vi "XY Graph Data Types.vi"() -> ()   [LabVIEW 2023]
doc: "Illustrates the various data types that the XY Graph accepts. Use the XY Graph to display data that is not uniformly distributed along the X-axis. This is particularly useful when displaying data that was sampled at a variable rate. The XY Graph is also useful for displaying data that is formatted as (X,Y) pairs."
panel:
  in  "Tab Control":T1(tab)
  out "Single Plot (Array of X,Y Pairs)":cluster{i32, dbl}[](graph)
  out "Multiple Plots (Array of X,Y Pairs)":cluster{cluster{i32, dbl}[]}[](graph)
  out "Single Plot (X Array and Y Array)":cluster{i32[], dbl[]}(graph)
  out "Multiple Plots (X Array and Y Array)":cluster{i32[], dbl[]}[](graph)
  # "Overview: Demonstrates various XY Graph data types.\nInstructions:\n1. Run the VI.\n2. Switch between the tabs to observe the appearance of the various XY Graphs."
  # "XY graphs that use (X,Y) pairs are arrays of clusters on the block diagram."
  # "XY graphs that use arrays of X values and arrays of Y values are clusters of arrays on the block diagram."
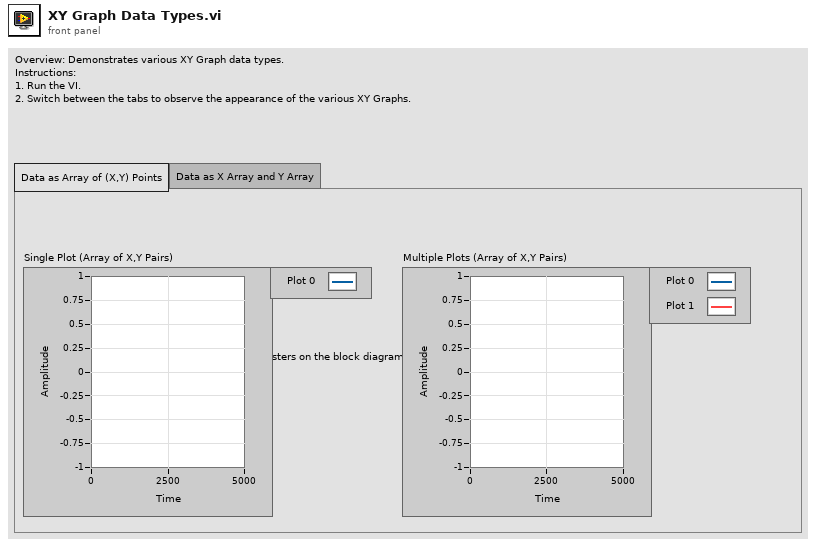
[diagram p1: front panel]
types:
  T1 = enum32{"Data as Array of (X,Y) Points", "Data as X Array and Y Array"}
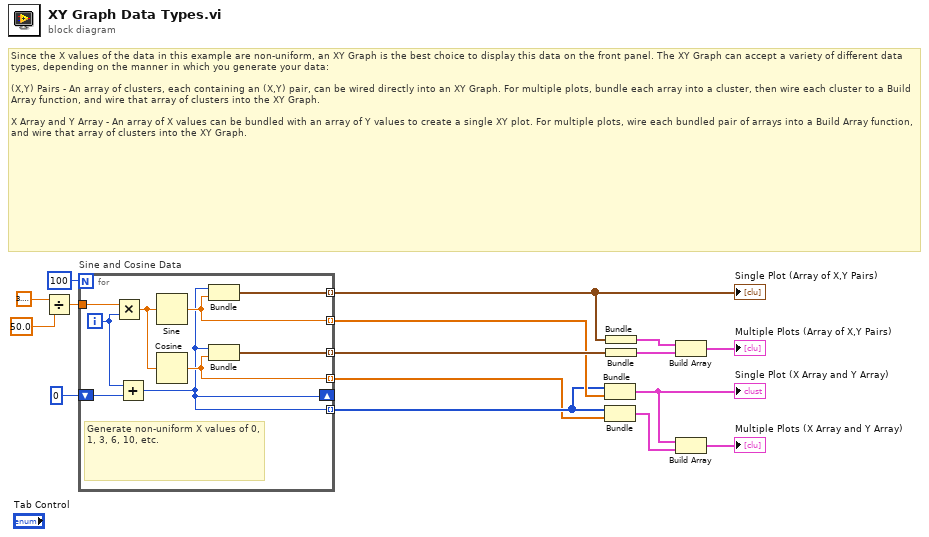
[diagram p0: block diagram]
diagram:
  # "Since the X values of the data in this example are non-uniform, an XY Graph is the best choice to display this data on the front panel. The XY Graph can accept a variety of different data types, depending on the manner in which you generate your data:\n\n(X,Y) Pairs - An array of clusters, each containing an (X,Y) pair, can be wired directly into an XY Graph. For multiple plots, bundle each array into a cluster, then wire each cluster to a Build Array function, and wire that array of clusters into the XY Graph.\n\nX Array and Y Array - An array of X values can be bundled with an array of Y values to create a single XY plot. For multiple plots, wire each bundled pair of arrays into a Build Array function, and wire that array of clusters into the XY Graph."
  n1 = Divide(x=3.141592653589793, y=50.0) -> (x/y=w14:dbl)
  n2 = for "Sine and Cosine Data" {
    N: 100 -> [_]
    tunnel: w14 -> [w25]
    tunnel: [w23] -> w6 mode=indexing
    tunnel: [w22] -> w4 mode=indexing
    shift-right: [w17] -> _
    shift-left: 0 -> [w21]
    tunnel: [w19] -> w10 mode=indexing
    tunnel: [w18] -> w11 mode=indexing
    tunnel: [w17] -> w5 mode=indexing
    i -> [w20]
    # "Generate non-uniform X values of 0, 1, 3, 6, 10, etc."
    n3 = Multiply(x=w25, y=w20) -> (x*y=w24:dbl)
    n4 = Add(x=w20, y=w21) -> (x+y=w17:i32)
    n5 = Sine(x=w24) -> (sin(x)=w23:dbl)
    n6 = Cosine(x=w24) -> (cos(x)=w22:dbl)
    n7 = Bundle(w17, w23) -> (w18:cluster{i32, dbl})  [unwired: 1 in]
    n8 = Bundle(w17, w22) -> (w19:cluster{i32, dbl})  [unwired: 1 in]
  }
  "Single Plot (Array of X,Y Pairs)" <- w11
  n9 = Bundle(w5, w6) -> (w3:cluster{i32[], dbl[]})  [unwired: 1 in]
  "Single Plot (X Array and Y Array)" <- w3
  n10 = Bundle(w5, w4) -> (w2:cluster{i32[], dbl[]})  [unwired: 1 in]
  n11 = Bundle(w11) -> (w7:cluster{cluster{i32, dbl}[]})  [unwired: 1 in]
  n12 = Bundle(w10) -> (w9:cluster{cluster{i32, dbl}[]})  [unwired: 1 in]
  n13 = Build Array(w7, w9) -> (→"Multiple Plots (Array of X,Y Pairs)":cluster{cluster{i32, dbl}[]}[])
  n14 = Build Array(w3, w2) -> (→"Multiple Plots (X Array and Y Array)":cluster{i32[], dbl[]}[])
